vi "Ripple tolerance.vi"(0 "Data Sample":dbl, 7 "Upper":string, 9 "Lower":string, 11 "error in (no error)":errorcluster) -> (4 "Boolean":bool, 15 "error out":errorcluster)   [LabVIEW 2018]
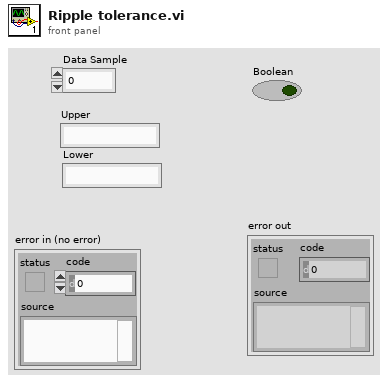
[diagram p1: front panel]
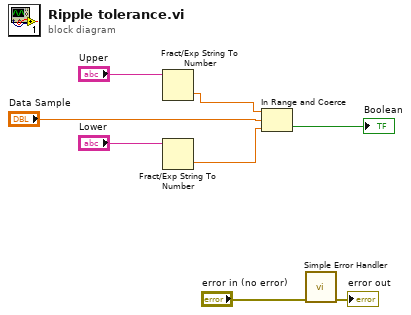
[diagram p0: block diagram]
diagram:
  n1 = Fract/Exp String To Number(string="Upper") -> (number=w4:dbl)  [unwired: 3 in, 1 out]
  n2 = Fract/Exp String To Number(string="Lower") -> (number=w3:dbl)  [unwired: 3 in, 1 out]
  n3 = In Range and Coerce(upper limit=w4, x="Data Sample", lower limit=w3) -> (In Range?=→"Boolean":bool)  [unwired: 1 out]
  n4 = call <vilib>:"Simple Error Handler.vi"("error in (no error)"="error in (no error)") -> ("error out"=→"error out":errorcluster)  [unwired: 4 in, 4 out]
